vi "Load Modules.vi"(8 "error in (no error)":errorcluster, 11 "Monitor-Pulse in":refnum<class "LabActor.lvclass">) -> (0 "error out":errorcluster, 3 "Monitor-Pulse out":refnum<class "LabActor.lvclass">)   [LabVIEW 2018, in "LabActor.lvclass"]
uses:
  LabActor.lvclass
  C:/github/2018/LabActor/Controllers/Application Controller/Application Controller.lvclass
  Controllers/Application Controller/Menu Control.ctl
  Controllers/Application Controller/Application Controller.lvclass/Application Controller.ctl
  Controllers/Pulse Controller/Pulse Controller.lvclass
  C:/github/2018/LabActor/Template Module/Template Module.lvclass
  Post-Processors/Integrate/Integrate.lvclass
  Post-Processors/Format Converter/Format Converter.lvclass
  Post-Processors/Lockin Processor/Lockin Processor.lvclass
  Controllers/Application Controller/Read Startup Configuration.vi
  Controllers/Application Controller/Application Controller.lvclass
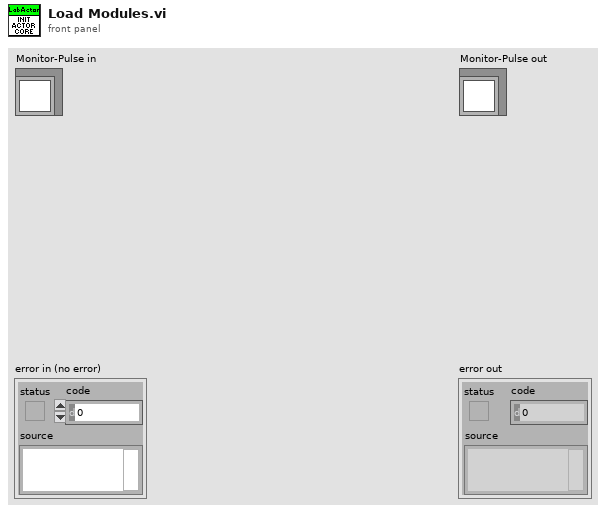
[diagram p1: front panel]
types:
  T1 = typedef "Menu Control.ctl" = enum16{"NONE", "Monitor", "Post-process", "Pulse"}
  T2 = typedef "Start-up Configuration.ctl" = cluster{"Load Modules":T3[], "External Modules Loaders":string[]}
  T3 = typedef "Module Types.ctl" = enum16{"NONE", "NI-DAQmx", "NI-Scope", "Red Pitaya Digitizer", "GaGe", "VISA Device", "Red Pitaya Lockin", "Monitor Controller", "Pulse Controller", "Integrate Pulse", "Lockin Processor", "File converter", "NHMFL Synthesizer", "Micron Hyperion", "Spectrum Recorder", "Resonance Detector", "TCP Communications", "Format Resonances", "Ruby Spectra", "PID Controller"}
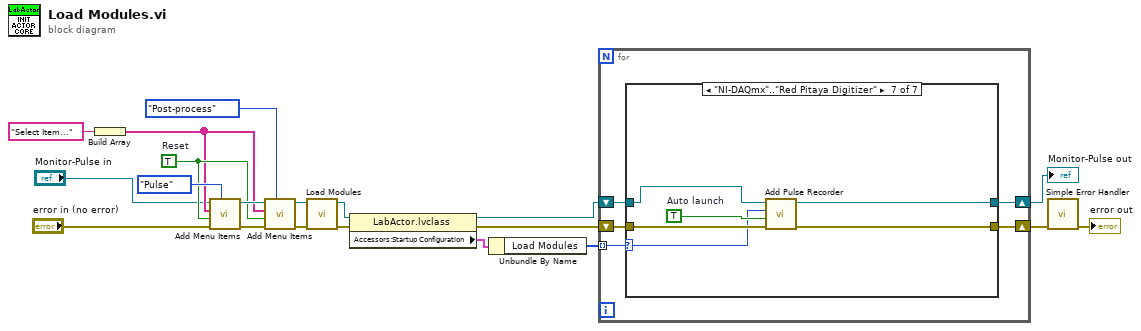
[diagram p0: block diagram]
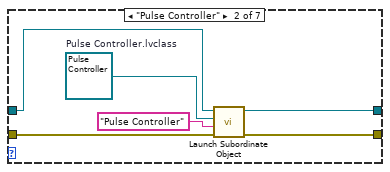
[diagram p3: hidden frame]
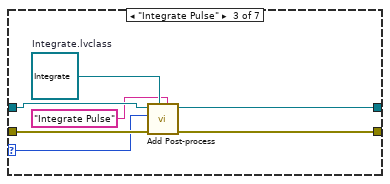
[diagram p4: hidden frame]
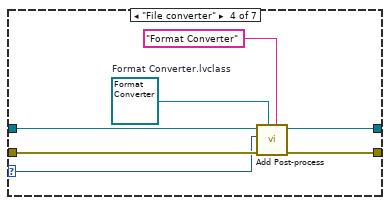
[diagram p5: hidden frame]
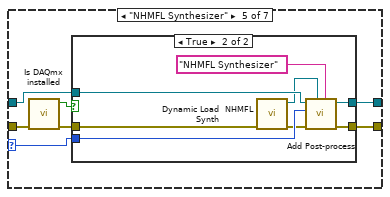
[diagram p6: hidden frame]
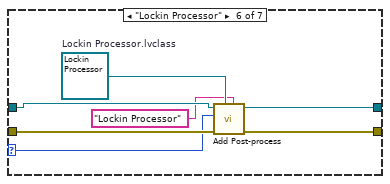
[diagram p8: hidden frame]
diagram:
  w14 = TRUE  # Reset
  n1 = Build Array("Select Item..." ("element")) -> (w13:string[])
  n2 = call-dynamic "Add Menu Items.vi"("Menu control"=Menu_Control."Pulse", "error in (no error)"="error in (no error)", "Reset"=w14, "Item Names"=w13, "Monitor-Pulse in"="Monitor-Pulse in") -> ("error out"=w18:errorcluster, "Monitor-Pulse out"=w19:refnum<class "LabActor.lvclass">)  [unwired: 5 in]
  n3 = call-dynamic "Add Menu Items.vi"("Menu control"=Menu_Control."Post-process", "error in (no error)"=w18, "Reset"=w14, "Item Names"=w13, "Monitor-Pulse in"=w19) -> ("error out"=w6:errorcluster, "Monitor-Pulse out"=w5:refnum<class "LabActor.lvclass">)  [unwired: 5 in]
  n4 = call-parent "Load Modules.vi"("error in (no error)"=w6, "Application Controller in"=w5) -> ("error out"=w4:errorcluster, "Application Controller out"=w3:refnum<class "LabActor.lvclass">)  [unwired: 8 in]
  n5 = property class="LabActor.lvclass"(reference=w3, error in=w4) -> (reference out=w11:refnum<class "LabActor.lvclass">, error out=w12:errorcluster, "Accessors:Startup Configuration"=w10:T2)
  n6 = Unbundle By Name(w10) -> ("Load Modules"=w9:T3[])
  n7 = for {
    tunnel: w9 -> [w25] mode=indexing
    shift-right: [w23] -> w1
    shift-left: w12 -> [w24]
    shift-right: [w22] -> w2
    shift-left: w11 -> [w21]
    n8 = case shown="\"NI-DAQmx\"..\"Red Pitaya Digitizer\"" w25 {
      selector: w25 -> [_ _ w34 w41 w51 w65 w72]
      tunnel: w24 -> [w26 w29 w36 w43 w50 w67 w74]
      tunnel: [w26 w28 w35 w42 w52 w66 w75] -> w23
      tunnel: w21 -> [w27 w31 w40 w47 w54 w71 w77]
      tunnel: [w27 w30 w39 w46 w53 w70 w76] -> w22
      frame "NONE", Default {
      }
      frame "Pulse Controller" {
        w32 = refnum<class "Pulse Controller.lvclass"> refnum  # Pulse Controller.lvclass
        n9 = call-dynamic "Launch Subordinate Object.vi"("error in (no error)"=w29, "Name"="Pulse Controller", "Subordinate Object"=w32, "Measure Object in"=w31) -> ("error out"=w28:errorcluster, "Measure Object out"=w30:refnum<class "LabActor.lvclass">)  [unwired: 5 in, 1 out]
      }
      frame "Integrate Pulse" {
        w38 = refnum<class "Integrate.lvclass"> refnum  # Integrate.lvclass
        n10 = call-dynamic "Add Post-process.vi"("Name"="Integrate Pulse", "Subordinate Object"=w38, "error in (no error)"=w36, "Module type"=w34, "Monitor-Pulse in"=w40) -> ("error out"=w35:errorcluster, "Monitor-Pulse out"=w39:refnum<class "LabActor.lvclass">)  [unwired: 5 in]
      }
      frame "File converter" {
        w45 = refnum<class "Format Converter.lvclass"> refnum  # Format Converter.lvclass
        n11 = call-dynamic "Add Post-process.vi"("Name"="Format Converter", "Subordinate Object"=w45, "error in (no error)"=w43, "Module type"=w41, "Monitor-Pulse in"=w47) -> ("error out"=w42:errorcluster, "Monitor-Pulse out"=w46:refnum<class "LabActor.lvclass">)  [unwired: 5 in]
      }
      frame "NHMFL Synthesizer" {
        n12 = call "Is DAQmx installed.vi"("Error In"=w50) -> ("Error Out"=w49:errorcluster, "file or folder exists?"=w48:bool)  [unwired: 9 in]
        n13 = case shown="True" w48 {
          tunnel: w54 -> [w56 w64]
          tunnel: [w56 w63] -> w53
          tunnel: [w55 w61] -> w52
          tunnel: w51 -> [_ w60]
          tunnel: w49 -> [w55 w59]
          frame False {
          }
          frame True {
            n14 = call "Dynamic Load  NHMFL Synth .vi"("Error In"=w59) -> ("Error Out"=w58:errorcluster, "Module"=w57:refnum<class "Template Module.lvclass">)  [unwired: 9 in]
            n15 = call-dynamic "Add Post-process.vi"("Name"="NHMFL Synthesizer", "Subordinate Object"=w57, "error in (no error)"=w58, "Module type"=w60, "Monitor-Pulse in"=w64) -> ("error out"=w61:errorcluster, "Monitor-Pulse out"=w63:refnum<class "LabActor.lvclass">)  [unwired: 5 in]
          }
        }
      }
      frame "Lockin Processor" {
        w69 = refnum<class "Lockin Processor.lvclass"> refnum  # Lockin Processor.lvclass
        n16 = call-dynamic "Add Post-process.vi"("Name"="Lockin Processor", "Subordinate Object"=w69, "error in (no error)"=w67, "Module type"=w65, "Monitor-Pulse in"=w71) -> ("error out"=w66:errorcluster, "Monitor-Pulse out"=w70:refnum<class "LabActor.lvclass">)  [unwired: 5 in]
      }
      frame "NI-DAQmx".."Red Pitaya Digitizer" {
        w73 = TRUE  # Auto launch
        n17 = call-dynamic "Add Pulse Recorder.vi"("error in (no error)"=w74, "Auto launch"=w73, "Module type"=w72, "LabActor in"=w77) -> ("error out"=w75:errorcluster, "LabActor out"=w76:refnum<class "LabActor.lvclass">)  [unwired: 6 in]
      }
    }
  }
  "Monitor-Pulse out" <- w2
  n18 = call <vilib>:"Simple Error Handler.vi"("error in (no error)"=w1) -> ("error out"=→"error out":errorcluster)  [unwired: 4 in, 4 out]
